vi "is AH bridgeVISA.vi"(8 "Error In":errorcluster, 11 "VISA resource name":refnum<visa-resource-name>) -> (0 "Error Out":errorcluster, 2 "is AH?":bool, 3 "VISA resource name out":refnum<visa-resource-name>)   [LabVIEW 2016]
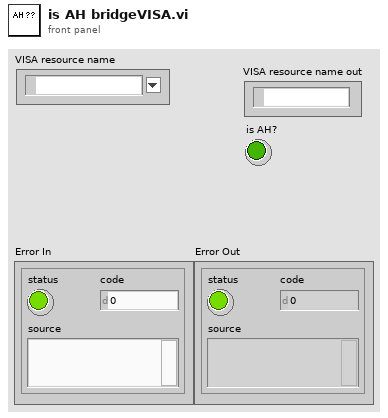
[diagram p1: front panel]
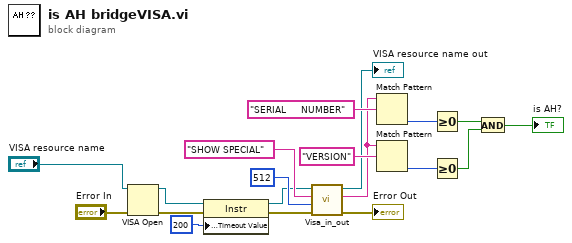
[diagram p0: block diagram]
diagram:
  n1 = VISA Open(error in (no error)="Error In", VISA resource name="VISA resource name") -> (VISA resource name=w9:refnum<visa-resource-name>, error out=w8:errorcluster)  [unwired: 3 in]
  n2 = property class="Instr"(reference=w9, error in=w8, "General Settings:Timeout Value"=u32 200) -> (reference out=w7:refnum<visa-resource-name>, error out=w6:errorcluster)
  n3 = call "Visa_in_out.vi"("error in (no error)"=w6, "read count"=u32 512, "write buffer"="SHOW SPECIAL", "VISA resource name"=w7) -> ("error out"=→"Error Out":errorcluster, "read buffer"=w12:string, "VISA resource name out"=→"VISA resource name out":refnum<visa-resource-name>)  [unwired: 5 in]
  n4 = Match Pattern(string=w12, regular expression="SERIAL     NUMBER") -> (offset past match=w16:i32)  [unwired: 1 in, 3 out]
  n5 = Match Pattern(string=w12, regular expression="VERSION") -> (offset past match=w13:i32)  [unwired: 1 in, 3 out]
  n6 = Greater Or Equal To 0?(x=w16) -> (x >= 0?=w15:bool)
  n7 = Greater Or Equal To 0?(x=w13) -> (x >= 0?=w11:bool)
  n8 = And(x=w15, y=w11) -> (x .and. y?=→"is AH?":bool)
